vi "Convert Write ERD List to Message (Rev 2 API).vi"(0 "GEA Inputs":T3 {"Destination" format="%.0x"; "Source" format="%.0x"}, 7 "ERD Read Data In":T1 {"ERD Number" format="%.0x"}, 11 "Error In":errorcluster) -> (4 "GEA Message":T4 {"Command" format="%02x"; "Destination" format="%02x"; "Source" format="%02x"}, 6 "Request ID":string, 15 "Error Out":errorcluster)   [LabVIEW 2023, in "GEA2_Toolkit.lvlib"]
doc: "This vi uses the Source / Destination from the GEA input and the ERD Write list to format a single GEA2 message to read the list of ERDs."
uses:
  library/GEA2_Toolkit.lvlib
  type defs/Data In.ctl
  type defs/Source_Destination.ctl
  type defs/ERD Write Data In.ctl
  type defs/Data Type.ctl
  <vilib>/regexp/Match Regular Expression.xnode
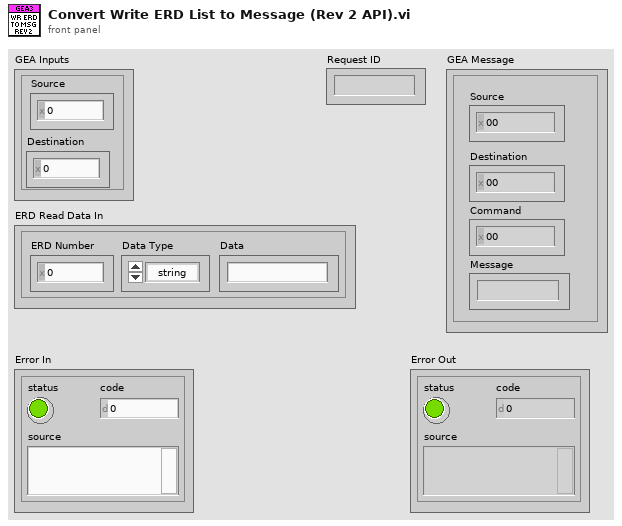
[diagram p1: front panel]
types:
  T1 = typedef "ERD Write Data In.ctl" = cluster{"ERD Number":u16, "Data Type":T2, "Data":string}
  T2 = typedef "Data Type.ctl" = enum16{"string", "boolean", "uint8_t", "uint16_t", "uint32_t", "uint64_t", "int8_t", "int16_t", "int32_t", "int64_t"}
  T3 = typedef "Source_Destination.ctl" = cluster{"Source":u8, "Destination":u8}
  T4 = typedef "Data In.ctl" = cluster{"Source":u8, "Destination":u8, "Command":u8, "Message":string}
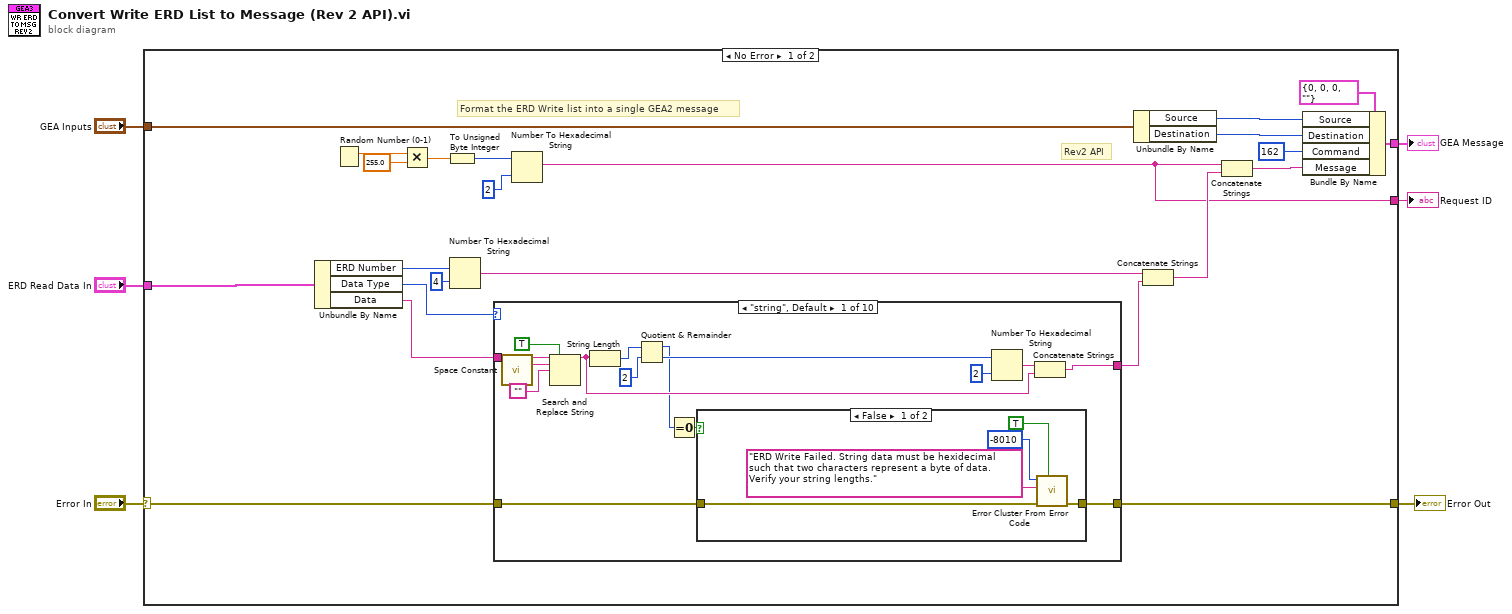
[diagram p0: block diagram]
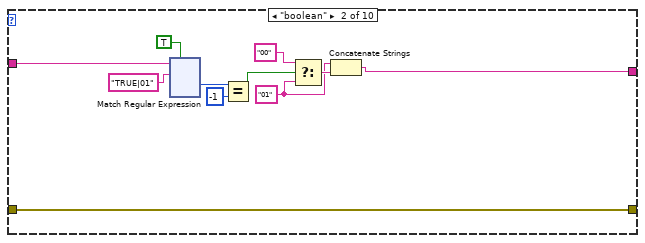
[diagram p3: hidden frame]
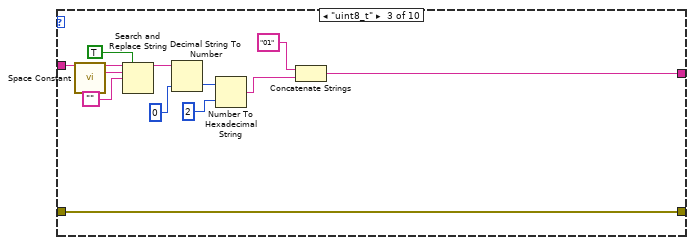
[diagram p4: hidden frame]
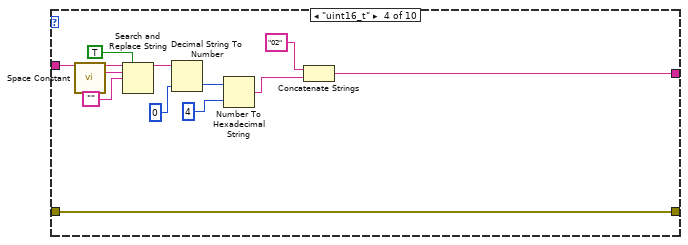
[diagram p5: hidden frame]
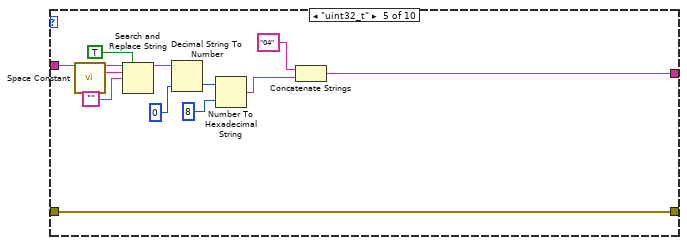
[diagram p6: hidden frame]
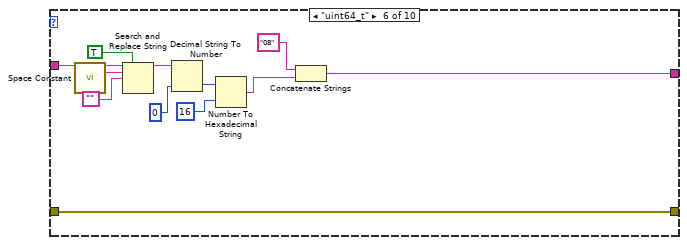
[diagram p7: hidden frame]
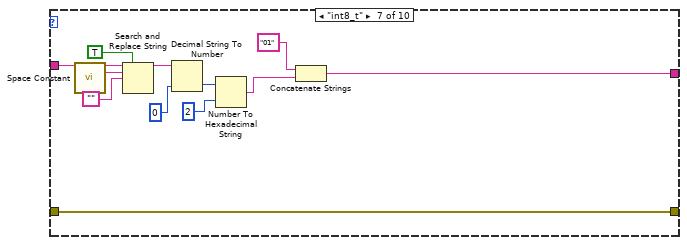
[diagram p8: hidden frame]
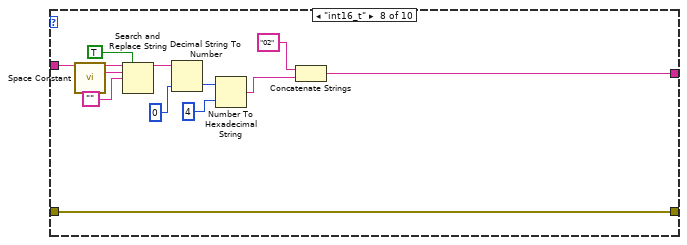
[diagram p9: hidden frame]
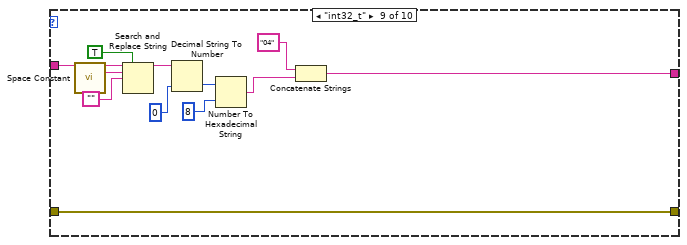
[diagram p10: hidden frame]
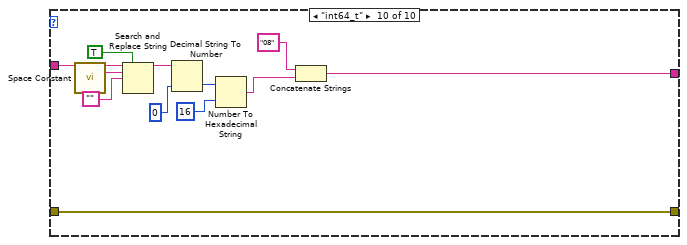
[diagram p11: hidden frame]
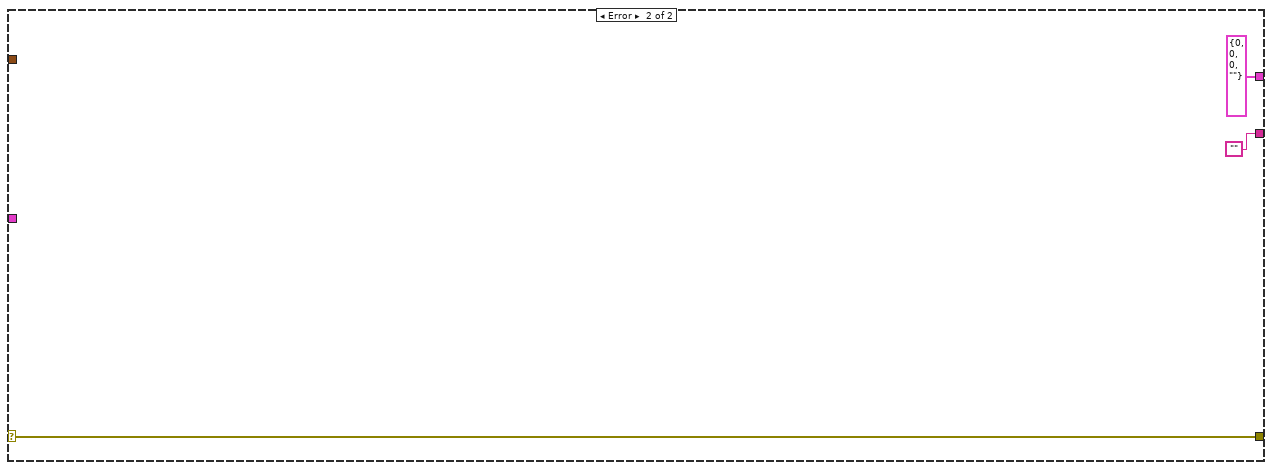
[diagram p12: hidden frame]
diagram:
  n1 = case shown="No Error" "Error In" {
    selector: "Error In" -> [w21 w277]
    tunnel: "GEA Inputs" -> [w27 _]
    tunnel: [w22 T4 {"Source"=0, "Destination"=0, "Command"=0, "Message"=""} ("GEA Message")] -> w5
    tunnel: [w20 w277] -> w3
    tunnel: [w8 ""] -> w2
    tunnel: "ERD Read Data In" -> [w7 _]
    frame No Error {
      # "Rev2 API"
      # "Format the ERD Write list into a single GEA2 message"
      n2 = Unbundle By Name(w7) -> ("ERD Number"=w19:u16, "Data Type"=w16:T2, "Data"=w15:string)
      n3 = Random Number (0-1)() -> (number: 0 to 1=w13:dbl)
      n4 = Multiply(x=w13, y=255.0) -> (x*y=w11:dbl)
      n5 = To Unsigned Byte Integer(number=w11) -> (unsigned 8bit integer=w10:u8)
      n6 = Number To Hexadecimal String(1:i16 4 ("width (-)"), 2:w19) -> (0:w17:string)
      n7 = case shown="\"string\", Default" w16 {
        tunnel: w15 -> [w44 w60 w187 w192 w205 w217 w229 w241 w253 w265]
        tunnel: [w39 w53 w186 w193 w204 w216 w228 w240 w252 w264] -> w14
        tunnel: w21 -> [w33 w51 w179 w191 w203 w215 w227 w239 w251 w263]
        tunnel: [w30 w51 w179 w191 w203 w215 w227 w239 w251 w263] -> w20
        frame "string", Default {
          n8 = call <vilib>:"Space Constant.vi"() -> ("String"=w42:string)
          n9 = Search and Replace String(replace all?=TRUE ("replace all? (F)"), input string=w44, search string=w42, replace string="") -> (result string=w38:string)  [unwired: 4 in, 3 out]
          n10 = String Length(string=w38) -> (length=w36:i32)
          n11 = Quotient & Remainder(x=w36, y=2) -> (x-y*floor(x/y)=w32:i32, floor(x/y)=w35:i32)
          n12 = Equal To 0?(x=w32) -> (x = 0?=w31:bool)
          n13 = case shown="False" w31 {
            tunnel: w33 -> [w49 w50]
            tunnel: [w45 w50] -> w30
            frame False {
              n14 = call <vilib>:"Error Cluster From Error Code.vi"("show call chain? (False)"=TRUE, "error in (no error)"=w49, "error message (\"\")"="ERD Write Failed. String data must be hexidecimal such that two characters represent a byte of data. Verify your string lengths." ("error message (\"\")"), "error code (0)"=-8010) -> ("error out"=w45:errorcluster)  [unwired: 5 in]
            }
            frame True {
            }
          }
          n15 = Number To Hexadecimal String(1:i16 2 ("width (-)"), 2:w35) -> (0:w40:string)
          n16 = Concatenate Strings(w40, w38) -> (w39:string)
        }
        frame "boolean" {
          w52 = "01"
          n17 = xnode "Match Regular Expression"("input string"=w60, "regular expression"="TRUE|01", "ignore case? (F)"=TRUE) -> ("offset past match"=w58:i32)  [unwired: 3 in, 4 out]
          n18 = Equal?(x=w58, y=-1) -> (x = y?=w55:bool)
          n19 = Select(t="00", s=w55, f=w52) -> (s? t:f=w54:string)
          n20 = Concatenate Strings(w52, w54) -> (w53:string)
        }
        frame "uint8_t" {
          n21 = call <vilib>:"Space Constant.vi"() -> ("String"=w189:string)
          n22 = Search and Replace String(replace all?=TRUE ("replace all? (F)"), input string=w187, search string=w189, replace string="") -> (result string=w184:string)  [unwired: 4 in, 3 out]
          n23 = Decimal String To Number(string=w184, default (0L)=u8 0) -> (number=w181:u8)  [unwired: 1 in, 1 out]
          n24 = Number To Hexadecimal String(1:i16 2 ("width (-)"), 2:w181) -> (0:w180:string)
          n25 = Concatenate Strings("01", w180) -> (w186:string)
        }
        frame "uint16_t" {
          n26 = call <vilib>:"Space Constant.vi"() -> ("String"=w201:string)
          n27 = Search and Replace String(replace all?=TRUE ("replace all? (F)"), input string=w192, search string=w201, replace string="") -> (result string=w198:string)  [unwired: 4 in, 3 out]
          n28 = Decimal String To Number(string=w198, default (0L)=u16 0) -> (number=w195:u16)  [unwired: 1 in, 1 out]
          n29 = Number To Hexadecimal String(1:i16 4 ("width (-)"), 2:w195) -> (0:w194:string)
          n30 = Concatenate Strings("02", w194) -> (w193:string)
        }
        frame "uint32_t" {
          n31 = call <vilib>:"Space Constant.vi"() -> ("String"=w213:string)
          n32 = Search and Replace String(replace all?=TRUE ("replace all? (F)"), input string=w205, search string=w213, replace string="") -> (result string=w210:string)  [unwired: 4 in, 3 out]
          n33 = Decimal String To Number(string=w210, default (0L)=u32 0) -> (number=w207:u32)  [unwired: 1 in, 1 out]
          n34 = Number To Hexadecimal String(1:i16 8 ("width (-)"), 2:w207) -> (0:w206:string)
          n35 = Concatenate Strings("04", w206) -> (w204:string)
        }
        frame "uint64_t" {
          n36 = call <vilib>:"Space Constant.vi"() -> ("String"=w225:string)
          n37 = Search and Replace String(replace all?=TRUE ("replace all? (F)"), input string=w217, search string=w225, replace string="") -> (result string=w222:string)  [unwired: 4 in, 3 out]
          n38 = Decimal String To Number(string=w222, default (0L)=u64 0) -> (number=w219:u64)  [unwired: 1 in, 1 out]
          n39 = Number To Hexadecimal String(1:i16 16 ("width (-)"), 2:w219) -> (0:w218:string)
          n40 = Concatenate Strings("08", w218) -> (w216:string)
        }
        frame "int8_t" {
          n41 = call <vilib>:"Space Constant.vi"() -> ("String"=w237:string)
          n42 = Search and Replace String(replace all?=TRUE ("replace all? (F)"), input string=w229, search string=w237, replace string="") -> (result string=w234:string)  [unwired: 4 in, 3 out]
          n43 = Decimal String To Number(string=w234, default (0L)=i8 0) -> (number=w231:i8)  [unwired: 1 in, 1 out]
          n44 = Number To Hexadecimal String(1:i16 2 ("width (-)"), 2:w231) -> (0:w230:string)
          n45 = Concatenate Strings("01", w230) -> (w228:string)
        }
        frame "int16_t" {
          n46 = call <vilib>:"Space Constant.vi"() -> ("String"=w249:string)
          n47 = Search and Replace String(replace all?=TRUE ("replace all? (F)"), input string=w241, search string=w249, replace string="") -> (result string=w246:string)  [unwired: 4 in, 3 out]
          n48 = Decimal String To Number(string=w246, default (0L)=i16 0) -> (number=w243:i16)  [unwired: 1 in, 1 out]
          n49 = Number To Hexadecimal String(1:i16 4 ("width (-)"), 2:w243) -> (0:w242:string)
          n50 = Concatenate Strings("02", w242) -> (w240:string)
        }
        frame "int32_t" {
          n51 = call <vilib>:"Space Constant.vi"() -> ("String"=w261:string)
          n52 = Search and Replace String(replace all?=TRUE ("replace all? (F)"), input string=w253, search string=w261, replace string="") -> (result string=w258:string)  [unwired: 4 in, 3 out]
          n53 = Decimal String To Number(string=w258, default (0L)=0) -> (number=w255:i32)  [unwired: 1 in, 1 out]
          n54 = Number To Hexadecimal String(1:i16 8 ("width (-)"), 2:w255) -> (0:w254:string)
          n55 = Concatenate Strings("04", w254) -> (w252:string)
        }
        frame "int64_t" {
          n56 = call <vilib>:"Space Constant.vi"() -> ("String"=w273:string)
          n57 = Search and Replace String(replace all?=TRUE ("replace all? (F)"), input string=w265, search string=w273, replace string="") -> (result string=w270:string)  [unwired: 4 in, 3 out]
          n58 = Decimal String To Number(string=w270, default (0L)=i64 0) -> (number=w267:i64)  [unwired: 1 in, 1 out]
          n59 = Number To Hexadecimal String(1:i16 16 ("width (-)"), 2:w267) -> (0:w266:string)
          n60 = Concatenate Strings("08", w266) -> (w264:string)
        }
      }
      n61 = Number To Hexadecimal String(1:i16 2 ("width (-)"), 2:w10) -> (0:w8:string)
      n62 = Unbundle By Name(w27) -> ("Source"=w26:u8, "Destination"=w25:u8)
      n63 = Concatenate Strings(w17, w14) -> (w29:string)
      n64 = Concatenate Strings(w8, w29) -> (w23:string)
      n65 = Bundle By Name(cluster=T4 {"Source"=0, "Destination"=0, "Command"=0, "Message"=""} ("GEA Message"), "Source"=w26, "Destination"=w25, "Command"=u8 162, "Message"=w23) -> (w22:T4)
    }
    frame Error {
    }
  }
  "GEA Message" <- w5
  "Error Out" <- w3
  "Request ID" <- w2
